vi "Coerce Port Power.vi"(0 "Cal Standard Base in":refnum<class "Cal Standard Base.lvclass">, 5 "Port Power":dbl, 11 "error in (no error)":errorcluster) -> (4 "Cal Standard Base out":refnum<class "Cal Standard Base.lvclass">, 6 "Coerced Port Power":dbl, 15 "error out":errorcluster)   [LabVIEW 2023, in "RFFixtureCharact.Instruments.lvlib" / "Cal Standard Base.lvclass"]
uses:
  Cal Standard Base.lvclass
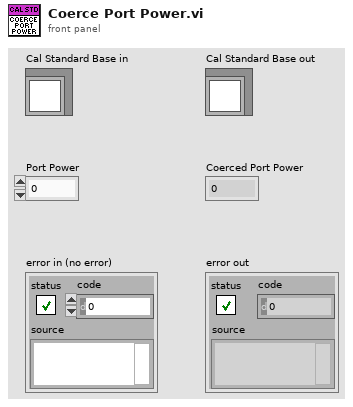
[diagram p1: front panel]
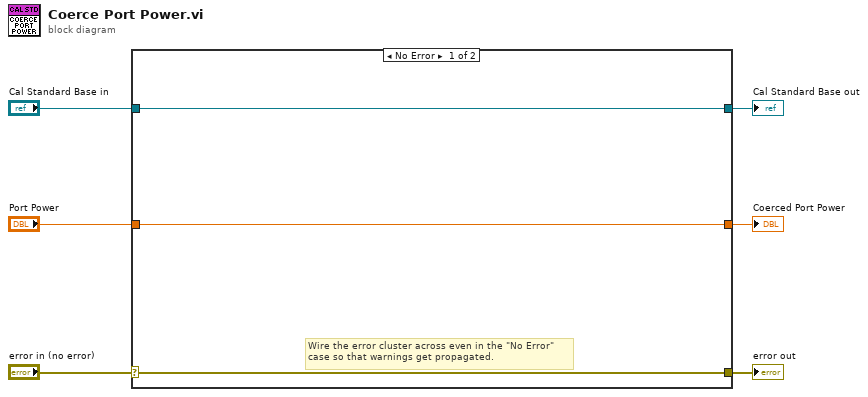
[diagram p0: block diagram]
diagram:
  n1 = case shown="No Error" "error in (no error)" {
    selector: "error in (no error)" -> [w8 w12]
    tunnel: [w8 w12] -> w5
    tunnel: [w9 w11] -> w3
    tunnel: "Cal Standard Base in" -> [w9 w11]
    tunnel: [w7 w10] -> w2
    tunnel: "Port Power" -> [w7 w10]
    frame No Error {
      # "Wire the error cluster across even in the \"No Error\"\ncase so that warnings get propagated."
    }
    frame Error {
    }
  }
  "error out" <- w5
  "Cal Standard Base out" <- w3
  "Coerced Port Power" <- w2
